vi "Relay Opt.vi"(8 "error in (no error)":errorcluster caption="错误输入（无错误）", 9 "OnOff":T1, 10 "Relay":T2, 11 "Input(U8)":u8 format="%.0x") -> (0 "error out":errorcluster caption="错误输出", 3 "Output(U8)":u8 format="%.0x")   [LabVIEW 2012]
uses:
  Relay Name.ctl
  OffOn.ctl
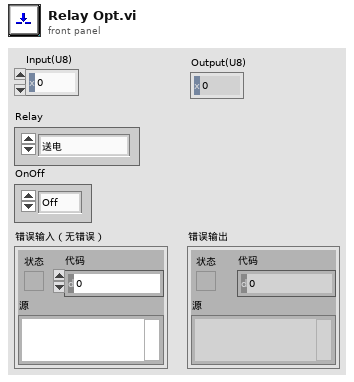
[diagram p1: front panel]
types:
  T1 = typedef "OffOn.ctl" = enum16{"Off", "On"}
  T2 = typedef "Relay Name.ctl" = enum8{"送电", "液压站", "润滑电机", "冷却电机", "滑台快进", "滑台工进", "滑台快退", "报警指示灯"}
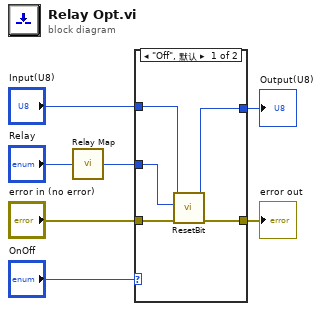
[diagram p0: block diagram]
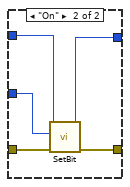
[diagram p2: hidden frame]
diagram:
  n1 = call "Relay Map.vi"("Relay"="Relay") -> ("bit"=w4:u8)  [unwired: 4 in]
  n2 = case shown="\"Off\", 默认" "OnOff" {
    tunnel: "Input(U8)" -> [w12 w17]
    tunnel: [w8 w16] -> w5
    tunnel: w4 -> [w11 w15]
    tunnel: "error in (no error)" -> [w10 w14]
    tunnel: [w9 w13] -> w2
    frame "Off", Default {
      n3 = call-poly "ResetBit.vi"("error in (no error)"=w10, "Bit(0-7)"=w11, "Input(U8)"=w12) -> ("error out"=w9:errorcluster, "Output(U8)"=w8:u8)  [unwired: 7 in]
    }
    frame "On" {
      n4 = call-poly "SetBit.vi"("error in (no error)"=w14, "Bit(0-7)"=w15, "Input(U8)"=w17) -> ("error out"=w13:errorcluster, "Output(U8)"=w16:u8)  [unwired: 7 in]
    }
  }
  "Output(U8)" <- w5
  "error out" <- w2
